vi "Client.vi"() -> ()   [LabVIEW 2018]
uses:
  Command_TypeDef.ctl
panel:
  in  "bytes to read":i32=100
  out "length":i32
  in  "Message":string="positionmirror ={\"command_name\": \"positionmirror\", \"unique_id\":2,\"command_data\":{\"private_rcvStamp\":1,\"x\":23,\"y\":21,\"z\":45,\"xRot\":34,\"yRot\":78,\"zRot\":98}}\n"
  in  "type":bool
  in  "Message Cluster":T1
  in  "stop":bool
  out "success":bool
  in  "send":bool
  in  "listening port":u16=50001
  in  "destination IP address":string="localhost"
  # "TCP Client"
  # "Cluster"
  # "String"
  # "restart VI after changing\nlistening port number"
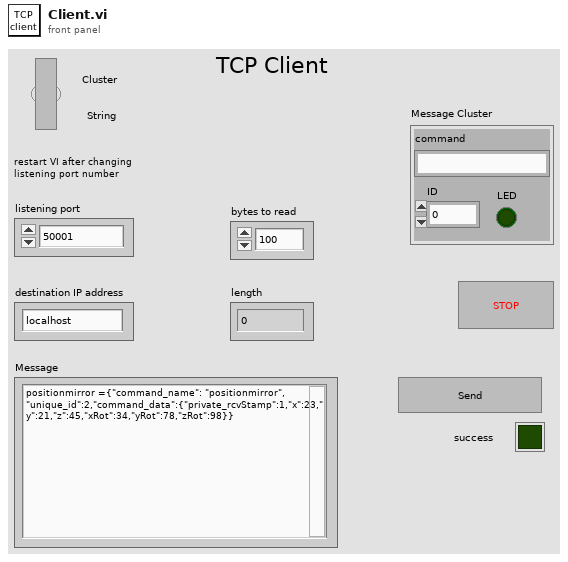
[diagram p1: front panel]
types:
  T1 = typedef "Command_TypeDef.ctl" = cluster{"command":string, "ID":i32, "LED":bool}
  T2 = enum16{"Standard", "Buffered", "CRLF", "Immediate"}
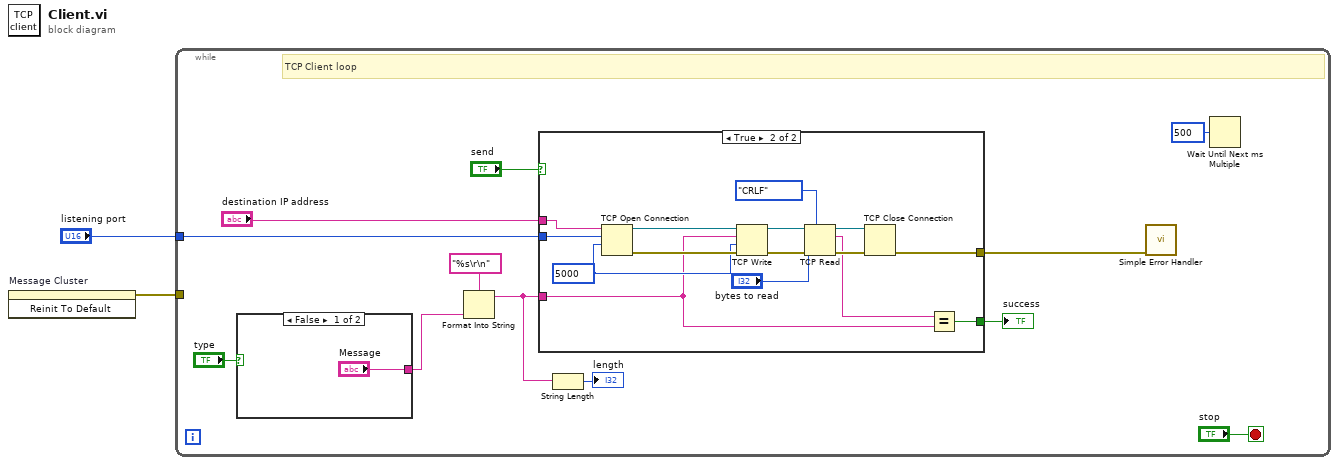
[diagram p0: block diagram]
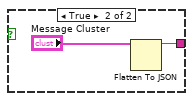
[diagram p2: hidden frame]
diagram:
  n1 = invoke on="Message Cluster" class="Clust (strict)" method="Reinit To Default"() -> (error out=w1:errorcluster)  [unwired: 3 in, 2 out]
  n2 = while {
    tunnel: "listening port" -> [w9]
    tunnel: w1 -> [_]
    stop <- "stop" stop-if-true
    # "TCP Client loop"
    n3 = case shown="False" "type" {
      tunnel: ["Message" w16] -> w7
      frame False {
      }
      frame True {
        n4 = Flatten To JSON(anything="Message Cluster") -> (JSON string=w16:string)  [unwired: 2 in, 1 out]
      }
    }
    n5 = Format Into String(format string="%s\r\n", w7) -> (resulting string=w5:string)  [unwired: 2 in, 1 out]
    n6 = case shown="True" "send" {
      tunnel: [_ w23] -> w12
      tunnel: w5 -> [_ w22]
      tunnel: "destination IP address" -> [_ w32]
      tunnel: w9 -> [_ w31]
      tunnel: [_ w19] -> w10
      frame False {
      }
      frame True {
        w28 = 5000 ("timeout ms (60000)")
        n7 = TCP Open Connection(address=w32, remote port or service name=w31, timeout ms (60000)=w28) -> (connection ID=w29:refnum<k5>, error out=w30:errorcluster)  [unwired: 2 in]
        n8 = TCP Write(connection ID=w29, data in=w22, error in (no error)=w30, 9:w28) -> (connection ID out=w27:refnum<k5>, error out=w26:errorcluster)  [unwired: 1 out]
        n9 = TCP Read(connection ID=w27, bytes to read="bytes to read", error in (no error)=w26, 7:T2."CRLF" ("mode (standard)")) -> (connection ID out=w24:refnum<k5>, data out=w20:string, error out=w25:errorcluster)  [unwired: 1 in]
        n10 = TCP Close Connection(connection ID=w24, error in (no error)=w25) -> (error out=w23:errorcluster)  [unwired: 1 in, 1 out]
        n11 = Equal?(x=w20, y=w22) -> (x = y?=w19:bool)
      }
    }
    "success" <- w10
    n12 = String Length(string=w5) -> (length=→"length":i32)
    n13 = call <vilib>:"Simple Error Handler.vi"("error in (no error)"=w12) -> ()  [unwired: 4 in, 5 out]
    n14 = Wait Until Next ms Multiple(millisecond multiple=u32 500) -> ()  [unwired: 1 out]
  }
